vi "fgv_Time series status.vi"(9 "Function":T1, 11 "Timelapse?":bool) -> (3 "Timelapse?":bool)   [LabVIEW 2017]
uses:
  Typedefs/Read Write Enum.ctl
  General Globals.vi
panel:
  # "SUBROUTINE"
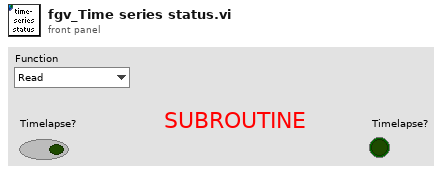
[diagram p1: front panel]
types:
  T1 = typedef "Read Write Enum.ctl" = enum16{"Read", "Write"}
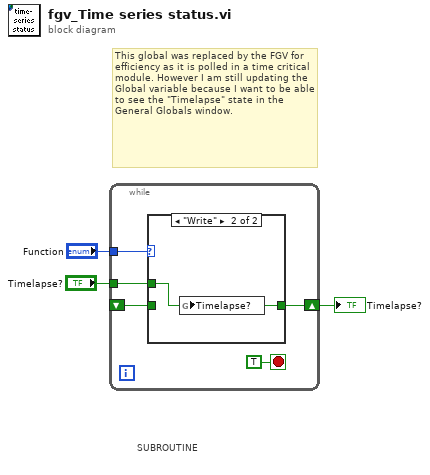
[diagram p0: block diagram]
diagram:
  # "SUBROUTINE"
  # "This global was replaced by the FGV for efficiency as it is polled in a time critical module. However I am still updating the Global variable because I want to be able to see the \"Timelapse\" state in the General Globals window."
  n1 = while {
    tunnel: "Function" -> [w7]
    tunnel: "Timelapse?" -> [w6]
    shift-right: [w5] -> w1
    shift-left: _ -> [w4]
    stop <- TRUE stop-if-true
    n2 = case shown="\"Write\"" w7 {
      tunnel: w6 -> [_ w10]
      tunnel: [w9 w10] -> w5
      tunnel: w4 -> [w9 _]
      frame "Read", Default {
      }
      frame "Write" {
        n3 = global write "General Globals.vi" "Timelapse?"(w10) -> ()
      }
    }
  }
  "Timelapse?" <- w1
